vi "Status Bar Example.vi"() -> ()   [LabVIEW 2020]
panel:
  in  "Status":i32(listbox)
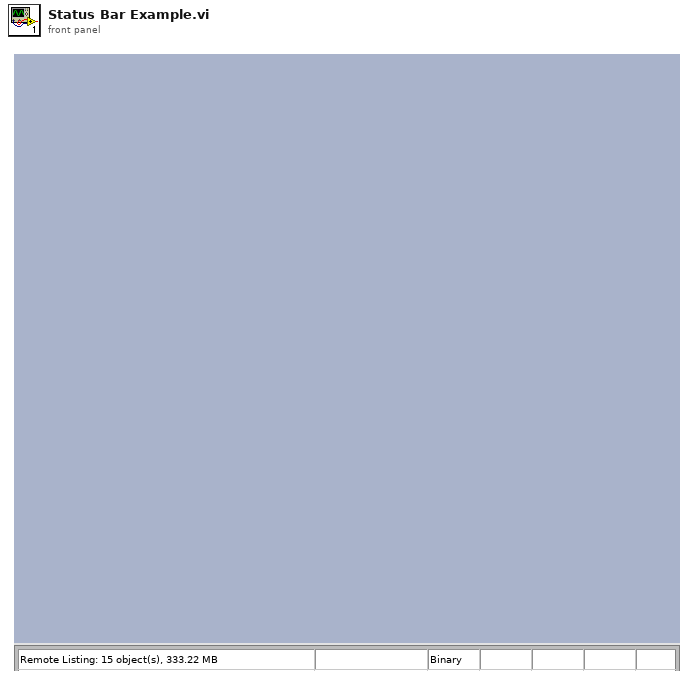
[diagram p1: front panel]
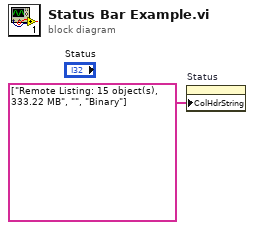
[diagram p0: block diagram]
diagram:
  n1 = property on="Status" class="MCListbox (strict)"("ColHdrString"=string[] ["Remote Listing: 15 object(s), 333.22 MB", "", "Binary"] ("Column Header Strings[]")) -> ()  [unwired: 2 in, 2 out]
